vi "Read waveform API.vi"(8 "Error In":errorcluster, 11 "Waveform name":string) -> (0 "Error Out":errorcluster)   [LabVIEW 2017, in "File IO.lvlib"]
uses:
  File IO.lvlib
  Controls/Command Data [cluster].ctl
  Controls/Commands [enum].ctl
  Events/Events.lvlib
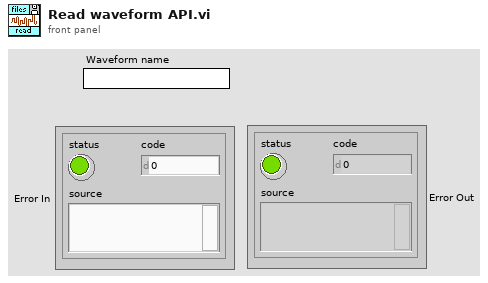
[diagram p1: front panel]
types:
  T1 = typedef "File IO.lvlib/Command Data [cluster].ctl" = cluster{"Command":T2, "Data":variant}
  T2 = typedef "File IO.lvlib/Commands [enum].ctl" = enum16{"Start", "Stop", "Read waveform", "Write waveform", "Delete waveform", "Log error", "Write config", "Read config", "Save parameters", "Send waveform to processing", "Update file prefix"}
  T3 = typedef "Events.lvlib/Refs [cluster].ctl" = cluster{"Exit":refnum<user-event>, "Controller":refnum<user-event>, "System Error":refnum<user-event>, "UI":refnum<user-event>, "Example Module":refnum<user-event>, "Shutter":refnum<user-event>, "Monochromator":refnum<user-event>, "DAQ":refnum<user-event>, "Scope":refnum<user-event>, "Processing":refnum<user-event>, "File IO":refnum<user-event>, "Colour wheel":refnum<user-event>}
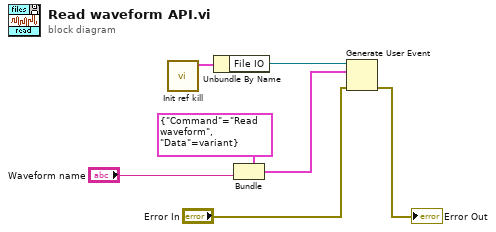
[diagram p0: block diagram]
diagram:
  n1 = call "Init ref kill.vi"() -> ("Messages"=w7:T3)  [unwired: 10 in, 1 out]
  n2 = Unbundle By Name(w7) -> ("File IO"=w6:refnum<user-event>)
  n3 = Bundle(cluster=T1 {"Command"=enum."Read waveform", "Data"=variant} ("event data"), "Data"="Waveform name") -> (w2:T1)  [unwired: 1 in]
  n4 = Generate User Event(user event=w6, event data cluster=w2, error in="Error In") -> (error out=→"Error Out":errorcluster)  [unwired: 1 in, 1 out]
